vi "SetGetBus.vi"(7 "Set (f)":bool, 11 "Bus.lvclass":refnum<class "Bus.lvclass">) -> (3 "Bus.lvclass":refnum<class "Bus.lvclass">)   [LabVIEW 2014, in "Bus.lvclass"]
uses:
  Bus.lvclass
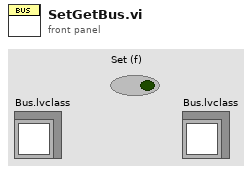
[diagram p1: front panel]
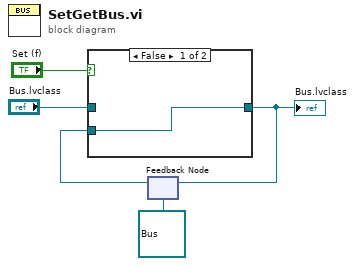
[diagram p0: block diagram]
diagram:
  n1 = feedback #1(refnum<class "Bus.lvclass"> refnum ("Bus.lvclass")) -> (w2:refnum<class "Bus.lvclass">)
  n2 = case shown="False" "Set (f)" {
    tunnel: "Bus.lvclass" -> [_ w7]
    tunnel: [w6 w7] -> w3
    tunnel: w2 -> [w6 _]
    frame False {
    }
    frame True {
    }
  }
  "Bus.lvclass" <- w3
  n3 = feedback-in #1(w3) -> ()
